vi "Command_Retract_Hatch.vi"(2 "Startup":bool) -> (3 "Reint":bool, 4 "Completed":bool, 5 "Press":T1)   [LabVIEW 2018]
uses:
  <vilib>/Rock Robotics/WPI/Solenoid/WPI_SolenoidValue.ctl
  Autonomous Utilities/Command_Execution_State.ctl
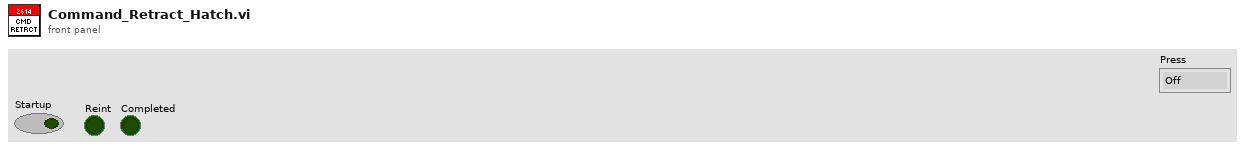
[diagram p1: front panel]
types:
  T1 = typedef "WPI_SolenoidValue.ctl" = enum16{"Off", "On", "Forward", "Reverse"}
  T2 = typedef "Command_Execution_State.ctl" = enum16{"Initialize", "Execute", "Finish"}
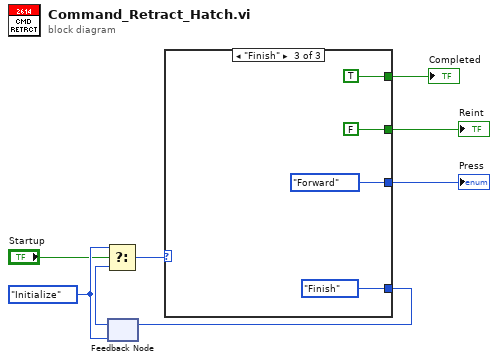
[diagram p0: block diagram]
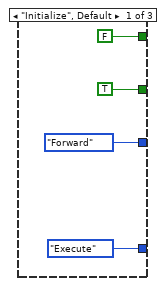
[diagram p2: hidden frame]
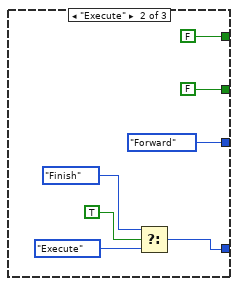
[diagram p3: hidden frame]
diagram:
  w5 = Command_Execution_State."Initialize" ("Play State")
  n1 = feedback #1(w5) -> (w6:T2)
  n2 = Select(t=w5, s="Startup", f=w6) -> (s? t:f=w8:T2)
  n3 = case shown="\"Finish\"" w8 {
    tunnel: [Command_Execution_State."Execute" ("Play State") w15 Command_Execution_State."Finish" ("Play State")] -> w7
    tunnel: [FALSE FALSE TRUE] -> w2
    tunnel: [TRUE FALSE FALSE] -> w3
    tunnel: [WPI_SolenoidValue."Forward" ("y") WPI_SolenoidValue."Forward" ("y") WPI_SolenoidValue."Forward" ("y")] -> w1
    frame "Initialize", Default {
    }
    frame "Execute" {
      n4 = Select(t=Command_Execution_State."Finish" ("Play State"), s=TRUE, f=Command_Execution_State."Execute" ("Play State")) -> (s? t:f=w15:T2)
    }
    frame "Finish" {
    }
  }
  "Reint" <- w3
  "Completed" <- w2
  "Press" <- w1
  n5 = feedback-in #1(w7) -> ()
